vi "Instrument Single Command.vi"(8 "Error In":errorcluster, 10 "Reset Command":string="*RST", 11 "VISA Name":string) -> (0 "Error Out":errorcluster)   [LabVIEW 2025]
doc: "Author: Scott Hannahs <sth@magnet.fsu.edu>\n\nThis software is licensed for use under the “MIT License\"\nCopyright (c) 2025 Scott Hannahs, sth@sth@magnet.sthnet.net\n\nPermission is hereby granted, free of charge, to any person obtaining a copy of this software and associated documentation files (the \"Software\"), to deal in the Software without restriction, including without limitation the rights to use, copy, modify, merge, publish, distribute, sublicense, and/or sell copies of the Software, and to permit persons to whom the Software is furnished to do so, subject to the following conditions: The above copyright notice and this permission notice shall be included in all copies or substantial portions of the Software.\n\nTHE SOFTWARE IS PROVIDED \"AS IS\", WITHOUT WARRANTY OF ANY KIND, EXPRESS OR IMPLIED, INCLUDING BUT NOT LIMITED TO THE WARRANTIES OF MERCHANTABILITY, FITNESS FOR A PARTICULAR PURPOSE AND NONINFRINGEMENT. IN NO EVENT SHALL THE AUTHORS OR COPYRIGHT HOLDERS BE LIABLE FOR ANY CLAIM, DAMAGES OR OTHER LIABILITY, WHETHER IN AN ACTION OF CONTRACT, TORT OR OTHERWISE, ARISING FROM, OUT OF OR IN CONNECTION WITH THE SOFTWARE OR THE USE OR OTHER DEALINGS IN THE SOFTWARE."
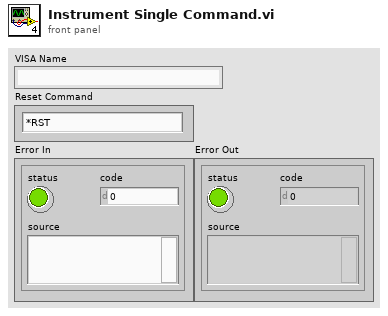
[diagram p1: front panel]
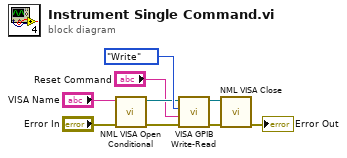
[diagram p0: block diagram]
diagram:
  n1 = call "NML VISA Open Conditional.vi"("error in (no error)"="Error In", "VISA resource name"="VISA Name") -> ("error out"=w3:errorcluster, "dup VISA Session"=w5:refnum<visa-resource-name>)  [unwired: 7 in, 1 out]
  n2 = call "VISA GPIB Write-Read.vi"("error in (no error)"=w3, "Command"="Reset Command", "Action"=enum16{"Write", "Read", "Write & Read"}."Write", "VISA resource name"=w5) -> ("error out"=w8:errorcluster, "dup VISA Session"=w9:refnum<visa-resource-name>)  [unwired: 4 in, 2 out]
  n3 = call "NML VISA Close.vi"("Error In"=w8, "VISA resource name"=w9) -> ("Error Out"=→"Error Out":errorcluster)  [unwired: 9 in]
